vi "AlliGator Get Simulation Options String.vi"(8 "Error In":errorcluster, 9 "Header Output":bool, 11 "Simulation & Fit Options & Parameters":T2 {"Decay Fit Options & Parameters"."Fit Options"."Confidence Level" min=0.0 max=100.0; "Decay Fit Options & Parameters"."Fit Options"."Offset Resolution" min=0.0; "Decay Fit Options & Parameters"."Fit Options"."Period" min=0.0; "Decay Fit Options & Parameters"."Fit Options"."Min Decay Percentile" min=0.0 max=1.0; "Decay Fit Options & Parameters"."Fit Options"."Max Decay Percentile" min=0.0 max=100.0; "Decay Fit Options & Parameters"."Fit Parameter Constraints"."Max Value" format="%#.3g"; "Decay Fit Options & Parameters"."Fit Parameter Constraints"."Min Value" format="%#.3g"}) -> (0 "Error Out":errorcluster, 1 "Simulation Output Header String":string, 2 "Fit Model":T1, 3 "Simulation Output String":string)   [LabVIEW 2021, in "AlliGator Fit Method Benchmark.lvlib"]
uses:
  AlliGator Fit Method Benchmark.lvlib
  AlliGator Simulation & Fit Options & Parameters.ctl
  AlliGator Simulation Parameters.ctl
  AlliGator Decay Simulation Parameters.ctl
  AlliGator Fit Simulation Parameters.ctl
  Decay Fit Parameter Map/AlliGator Decay Fit Options & Parameters v3.ctl
  Fits/IRF(X)PSED/Decay Fit Options v3.ctl
  Fits/Decay Convolution/Decay Model.ctl
  Fits/Residual Type.ctl
  Fits/IRF(X)PSED/Fit Weights Type.ctl
  Fits/Non-linear Fitting Method v2.ctl
  Fits/Fit Calculation Method.ctl
  Fits/Non-linear Fitting Algorithm.ctl
  Decay Analysis/Decay Fit/AlliGator Decay Fit Parameter Constraints 2.ctl
  Fits/IRF(X)PSED/Decay Fit Parameters In List.ctl
  Fits/IRF(X)PSED/MLE Baseline Offset Type.ctl
  Fits/Fits.lvlib
  Decay Analysis/Decay Fit/AlliGator Decay Fit.lvlib
  Decay Fit Parameter Map/AlliGator Decay Fit Parameter Map.lvlib
panel:
  # "see the License on the block diagram (Ctrl+E or Window:Show Block Diagram)"
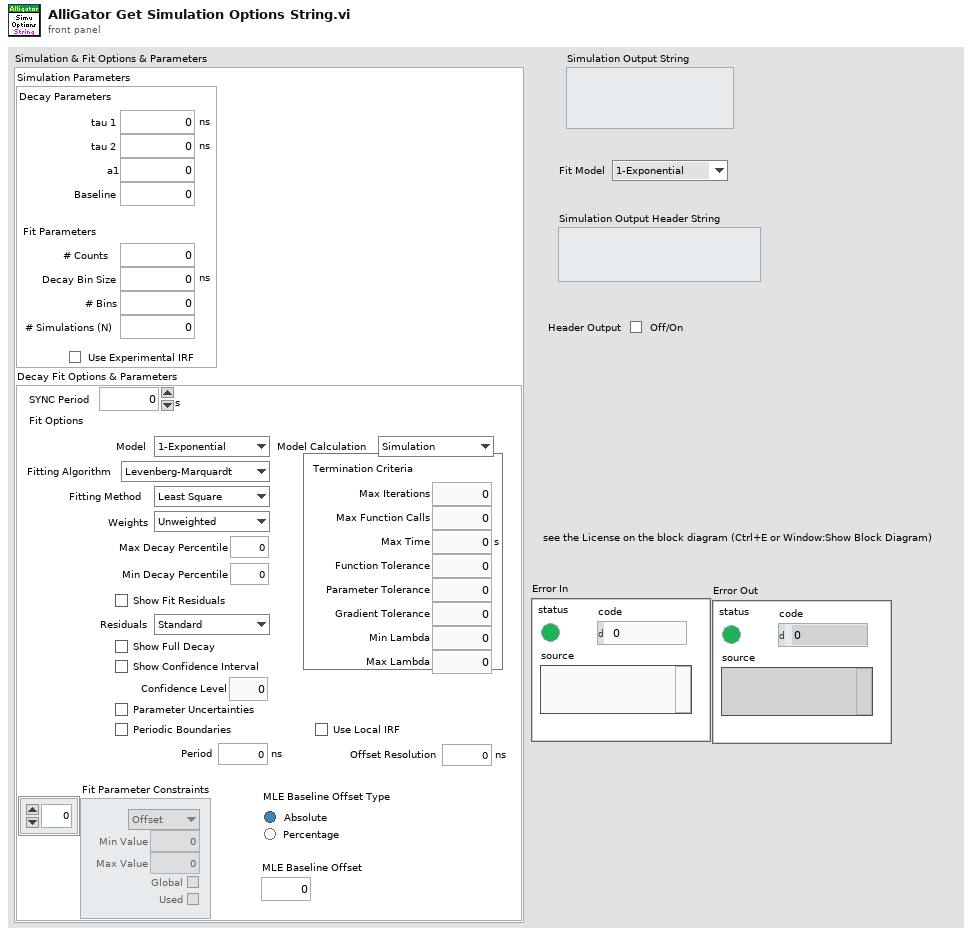
[diagram p1: front panel]
types:
  T1 = typedef "Fits.lvlib/Decay Model.ctl" = enum16{"1-Exponential", "2-Exponentials"}
  T2 = typedef "AlliGator Fit Method Benchmark.lvlib/AlliGator Simulation & Fit Options & Parameters.ctl" = cluster{"Simulation Parameters":T3, "Decay Fit Options & Parameters":T6}
  T3 = typedef "AlliGator Fit Method Benchmark.lvlib/AlliGator Simulation Parameters.ctl" = cluster{"Decay Simulation Parameters":T4, "Fit Simulation Parameters":T5, "Use Experimental IRF":bool}
  T4 = typedef "AlliGator Fit Method Benchmark.lvlib/AlliGator Decay Simulation Parameters.ctl" = cluster{"tau 1":dbl[unit], "tau 2":dbl[unit], "a1":dbl, "Baseline":dbl}
  T5 = typedef "AlliGator Fit Method Benchmark.lvlib/AlliGator Fit Simulation Parameters.ctl" = cluster{"# Counts":i32, "# Simulations (N)":i32, "Decay Bin Size":dbl[unit], "# Bins":i32}
  T6 = typedef "AlliGator Decay Fit Parameter Map.lvlib/AlliGator Decay Fit Options & Parameters v3.ctl" = cluster{"SYNC Period":dbl[unit], "Fit Options":T7, "Fit Parameter Constraints":T13[], "MLE Baseline Offset":dbl, "MLE Baseline Offset Type":T15}
  T7 = typedef "Fits.lvlib/Decay Fit Options v3.ctl" = cluster{"Show Fit Residuals":bool, "Fit Model":T1, "Residual Type":T8, "Max Decay Percentile":dbl, "Min Decay Percentile":dbl, "Show Full Decay":bool, "Weights":T9, "Fitting Method":T10, "Compute Parameter Uncertainties":bool, "Periodic Boundaries":bool, "Model Calculation":T11, "Period":dbl[unit], "Termination Criteria":cluster{"Max Iterations":i32, "Max Function Calls":i32, "Max Time":dbl[unit], "Function Tolerance":dbl, "Parameter Tolerance":dbl, "Gradient Tolerance":dbl, "Min Lambda":dbl, "Max Lambda":dbl, "Initial Tick Count":u32}, "Offset Resolution":dbl[unit], "Use Local IRF":bool, "Fitting Algorithm":T12, "Show Confidence Interval ":bool, "Confidence Level":dbl}
  T8 = typedef "Fits.lvlib/Residual Type.ctl" = enum16{"Standard", "Normalized", "Reduced"}
  T9 = typedef "Fits.lvlib/Fit Weights Type.ctl" = enum16{"Unweighted", "1/Variance", "Best of All"}
  T10 = typedef "Fits.lvlib/Non-linear Fitting Method v2.ctl" = enum16{"Least Square", "Least Absolute Residual", "Bisquare", "MLE", "-", "Best of All"}
  T11 = typedef "Fits.lvlib/Fit Calculation Method.ctl" = enum16{"Simulation", "Convolution", "Integration"}
  T12 = typedef "Fits.lvlib/Non-linear Fitting Algorithm.ctl" = enum16{"Levenberg-Marquardt", "Trust-Region Dogleg"}
  T13 = typedef "AlliGator Decay Fit.lvlib/AlliGator Decay Fit Parameter Constraints 2.ctl" = cluster{"Fit Parameter":T14, "Min Value":dbl, "Max Value":dbl, "Global":bool, "Used":bool}
  T14 = typedef "Fits.lvlib/Decay Fit Parameters In List.ctl" = enum16{"Offset", "Baseline", "A_1", "tau_1", "A_2", "tau_2"}
  T15 = typedef "Fits.lvlib/MLE Baseline Offset Type.ctl" = enum32{"Absolute", "Percentage"}
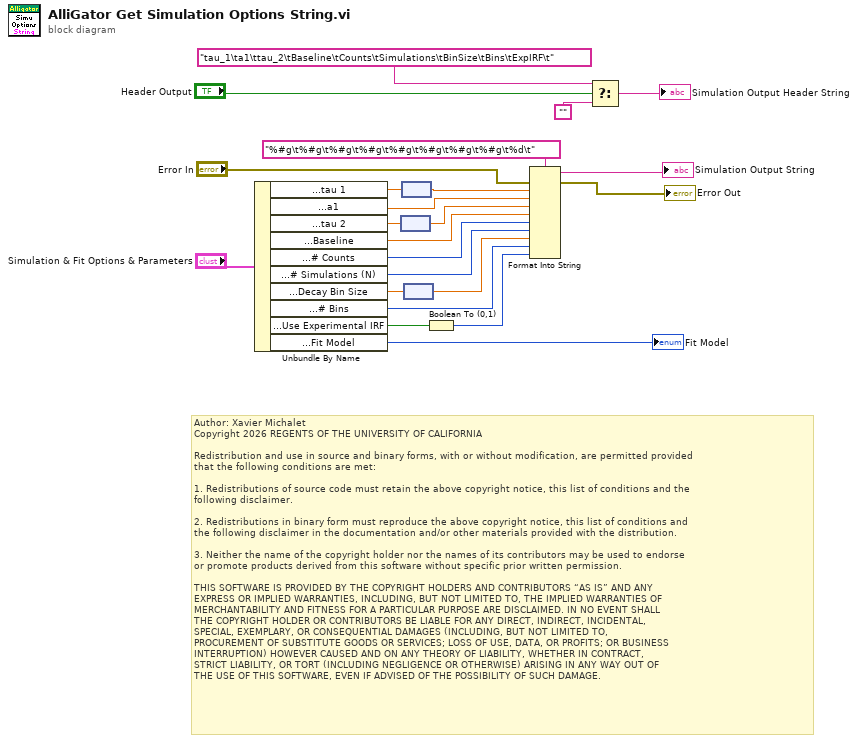
[diagram p0: block diagram]
diagram:
  # "Author: Xavier Michalet\nCopyright 2026 REGENTS OF THE UNIVERSITY OF CALIFORNIA\n\nRedistribution and use in source and binary forms, with or without modification, are permitted provided\nthat the following conditions are met:\n\n1. Redistributions of source code must retain the above copyright notice, this list of conditions and the\nfollowing disclaimer.\n\n2. Redistributions in binary form must reproduce the above copyright notice, this list of conditions and\nthe following disclaimer in the documentation and/or other materials provided with the distribution.\n\n3. Neither the name of the copyright holder nor the names of its contributors may be used to endorse \nor promote products derived from this software without specific prior written permission.\n\nTHIS SOFTWARE IS PROVIDED BY THE COPYRIGHT HOLDERS AND CONTRIBUTORS “AS IS” AND ANY \nEXPRESS OR IMPLIED WARRANTIES, INCLUDING, BUT NOT LIMITED TO, THE IMPLIED WARRANTIES OF\nMERCHANTABILITY AND FITNESS FOR A PARTICULAR PURPOSE ARE DISCLAIMED. IN NO EVENT SHALL\nTHE COPYRIGHT HOLDER OR CONTRIBUTORS BE LIABLE FOR ANY DIRECT, INDIRECT, INCIDENTAL, \nSPECIAL, EXEMPLARY, OR CONSEQUENTIAL DAMAGES (INCLUDING, BUT NOT LIMITED TO, \nPROCUREMENT OF SUBSTITUTE GOODS OR SERVICES; LOSS OF USE, DATA, OR PROFITS; OR BUSINESS\nINTERRUPTION) HOWEVER CAUSED AND ON ANY THEORY OF LIABILITY, WHETHER IN CONTRACT, \nSTRICT LIABILITY, OR TORT (INCLUDING NEGLIGENCE OR OTHERWISE) ARISING IN ANY WAY OUT OF\nTHE USE OF THIS SOFTWARE, EVEN IF ADVISED OF THE POSSIBILITY OF SUCH DAMAGE."
  n1 = Unbundle By Name("Simulation & Fit Options & Parameters") -> ("Simulation Parameters.Decay Simulation Parameters.tau 1"=w22:dbl[unit], "Simulation Parameters.Decay Simulation Parameters.a1"=w21:dbl, "Simulation Parameters.Decay Simulation Parameters.tau 2"=w20:dbl[unit], "Simulation Parameters.Decay Simulation Parameters.Baseline"=w19:dbl, "Simulation Parameters.Fit Simulation Parameters.# Counts"=w14:i32, "Simulation Parameters.Fit Simulation Parameters.# Simulations (N)"=w13:i32, "Simulation Parameters.Fit Simulation Parameters.Decay Bin Size"=w12:dbl[unit], "Simulation Parameters.Fit Simulation Parameters.# Bins"=w11:i32, "Simulation Parameters.Use Experimental IRF"=w10:bool, "Decay Fit Options & Parameters.Fit Options.Fit Model"=→"Fit Model":T1)
  n2 = node(w20) -> (w3:dbl)
  n3 = node(w22) -> (w4:dbl)
  n4 = node(w12) -> (w2:dbl)
  n5 = Boolean To (0,1)(Boolean=w10) -> (0, 1=w9:i16)
  n6 = Format Into String(format string="%#g\t%#g\t%#g\t%#g\t%#g\t%#g\t%#g\t%#g\t%d\t" ("Array Statistics Header String"), error in="Error In", w4, w21, w3, w19, w14, w13, w2, w11, w9) -> (resulting string=→"Simulation Output String":string, error out=→"Error Out":errorcluster)  [unwired: 1 in]
  n7 = Select(t="tau_1\ta1\ttau_2\tBaseline\tCounts\tSimulations\tBinSize\tBins\tExpIRF\t" ("Array Statistics Header String"), s="Header Output", f="") -> (s? t:f=→"Simulation Output Header String":string)
